vi "MattesImageRegistration.vi"(6 "Registration parameters":T1={"Sampling Percentage"=0.2, "maximum iteration"=200, "number of bins"=200}, 8 "error in (no error)":errorcluster, 9 "False color image in":T2, 10 "Moving image in":T2=refnum, 11 "Fixed image in":T2=refnum) -> (0 "error out":errorcluster, 1 "False color alignment image":T2, 2 "Moving image out (duplicate)":T2, 3 "Fixed image out (duplicate)":T2, 4 "alignment quality":dbl=-0.39635115330155946, 5 "y translation":dbl=4.5810062720041405, 7 "x translation":dbl=-23.66339978067731)   [LabVIEW 2012]
uses:
  <vilib>/vision/Image Controls.llb/IMAQ Image.ctl
  <vilib>/vision/NI_Vision_Development_Module.lvlib
  C++/bin/Release/ImageReg.dll
panel:
  out "elapsed time (ms)":u32=741
  out "# of iterations":dbl=100.0
  out "False color image":T2(plugin-control)
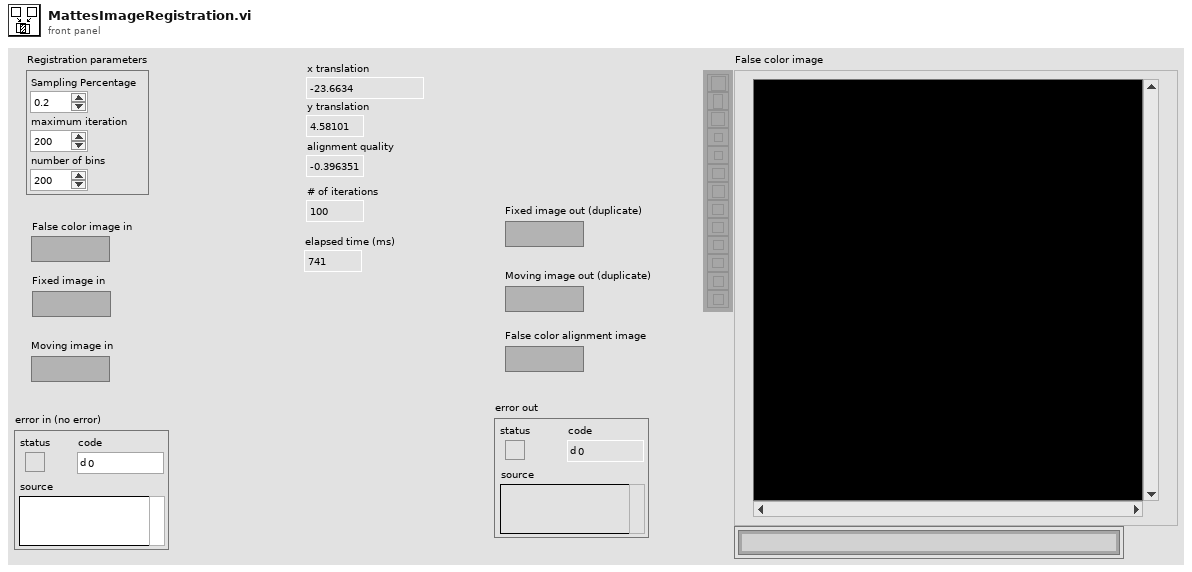
[diagram p1: front panel]
types:
  T1 = cluster{"Sampling Percentage":dbl, "maximum iteration":i32, "number of bins":u32}
  T2 = typedef "IMAQ Image.ctl" = refnum<image>
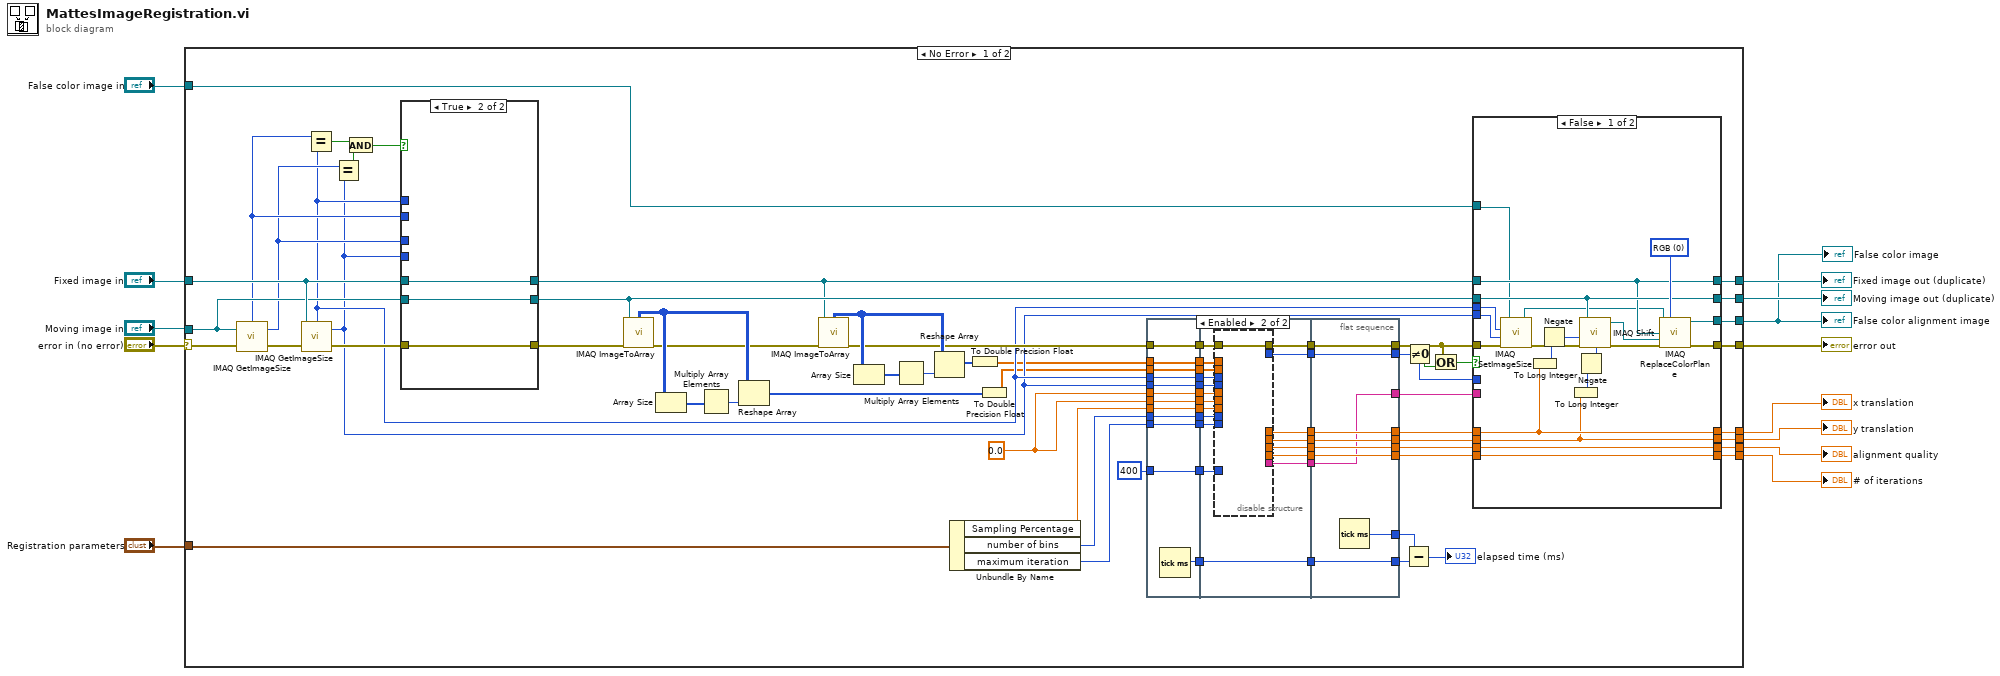
[diagram p0: block diagram]
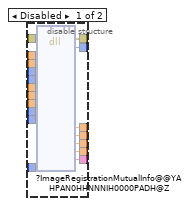
[diagram p2: hidden frame]
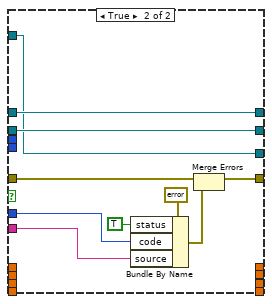
[diagram p3: hidden frame]
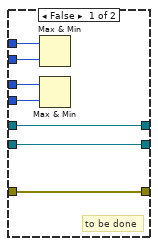
[diagram p4: hidden frame]
diagram:
  n1 = case shown="No Error" "error in (no error)" {
    selector: "error in (no error)" -> [w87 w191]
    tunnel: [w74 w191] -> w12
    tunnel: "Moving image in" -> [w81 w189]
    tunnel: "Fixed image in" -> [w82 w190]
    tunnel: [w67 _] -> w9
    tunnel: [w66 _] -> w8
    tunnel: [w65 _] -> w7
    tunnel: [w64 w188] -> w4
    tunnel: [w63 w189] -> w6
    tunnel: [w62 w190] -> w5
    tunnel: [w61 _] -> w3
    tunnel: "False color image in" -> [w30 w188]
    tunnel: "Registration parameters" -> [w27 _]
    frame No Error {
      w19 = 0.0 ("double precision float")
      n2 = call "IMAQ GetImageSize"("Image"=w81, "error in (no error)"=w87) -> ("Y Resolution"=w79:i32, "X Resolution"=w80:i32, "error out"=w86:errorcluster)  [unwired: 2 in]
      n3 = call "IMAQ GetImageSize"("Image"=w82, "error in (no error)"=w86) -> ("Y Resolution"=w57:i32, "X Resolution"=w58:i32, "error out"=w78:errorcluster)  [unwired: 2 in]
      n4 = Equal?(x=w80, y=w58) -> (x = y?=w84:bool)
      n5 = Equal?(x=w79, y=w57) -> (x = y?=w85:bool)
      n6 = And(x=w84, y=w85) -> (x .and. y?=w83:bool)
      n7 = case shown="True" w83 {
        tunnel: [w180 w187] -> w28
        tunnel: w82 -> [w180 w187]
        tunnel: [w179 w186] -> w29
        tunnel: w81 -> [w179 w186]
        tunnel: w58 -> [w184 _]
        tunnel: w80 -> [w183 _]
        tunnel: w79 -> [w182 _]
        tunnel: w57 -> [w181 _]
        tunnel: [w178 w185] -> w18
        tunnel: w78 -> [w178 w185]
        frame False {
          # "to be done"
          n8 = Max & Min(x=w184, y=w183) -> ()  [unwired: 2 out]
          n9 = Max & Min(x=w182, y=w181) -> ()  [unwired: 2 out]
        }
        frame True {
        }
      }
      n10 = call "IMAQ ImageToArray"("error in (no error)"=w18, "Image"=w29) -> ("error out"=w17:errorcluster, "Image Pixels (U8)"=w73:u8[][])  [unwired: 2 in, 3 out]
      n11 = Array Size(array=w73) -> (size(s)=w72:i32[])
      n12 = Multiply Array Elements(1:w72) -> (0:w71:i32)
      n13 = Reshape Array(w73, w71) -> (w77:u8[])
      n14 = call "IMAQ ImageToArray"("error in (no error)"=w17, "Image"=w28) -> ("error out"=w60:errorcluster, "Image Pixels (U8)"=w68:u8[][])  [unwired: 2 in, 3 out]
      n15 = Array Size(array=w68) -> (size(s)=w70:i32[])
      n16 = Multiply Array Elements(1:w70) -> (0:w69:i32)
      n17 = Reshape Array(w68, w69) -> (w21:u8[])
      n18 = Unbundle By Name(w27) -> ("Sampling Percentage"=w26:dbl, "number of bins"=w25:u32, "maximum iteration"=w16:i32)
      n19 = To Double Precision Float(number=w21) -> (double precision float=w20:dbl[])
      n20 = To Double Precision Float(number=w77) -> (double precision float=w22:dbl[])
      n21 = flat-sequence {
        tunnel: w26 -> [w92]
        tunnel: w19 -> [w93]
        tunnel: w19 -> [w94]
        tunnel: w57 -> [w95]
        tunnel: w58 -> [w96]
        tunnel: w22 -> [w97]
        tunnel: w20 -> [w98]
        tunnel: w60 -> [w99]
        tunnel: [w99] -> w51
        tunnel: [w98] -> w50
        tunnel: [w97] -> w49
        tunnel: [w96] -> w48
        tunnel: [w95] -> w47
        tunnel: [w94] -> w46
        tunnel: [w93] -> w45
        tunnel: [w92] -> w44
        tunnel: [w91] -> w36
        tunnel: [w90] -> w32
        tunnel: w16 -> [w90]
        tunnel: [w89] -> w31
        tunnel: w25 -> [w89]
        tunnel: 400 ("dimension size") -> [w88]
        tunnel: [w88] -> w14
        tunnel: w51 -> [w118]
        tunnel: w50 -> [w116]
        tunnel: w49 -> [w115]
        tunnel: w48 -> [w114]
        tunnel: w47 -> [w113]
        tunnel: w46 -> [w112]
        tunnel: w45 -> [w111]
        tunnel: w44 -> [w110]
        tunnel: [w117] -> w43
        tunnel: [w109] -> w42
        tunnel: [w108] -> w41
        tunnel: [w107] -> w40
        tunnel: [w106] -> w39
        tunnel: [w105] -> w38
        tunnel: w36 -> [w104]
        tunnel: [w104] -> w35
        tunnel: w32 -> [w103]
        tunnel: w31 -> [w102]
        tunnel: [w101] -> w23
        tunnel: w14 -> [w100]
        tunnel: [w141] -> w52
        tunnel: [w142] -> w53
        tunnel: [w143] -> w54
        tunnel: [w144] -> w55
        tunnel: [w145] -> w56
        tunnel: [w146] -> w59
        tunnel: w43 -> [w146]
        tunnel: w42 -> [w145]
        tunnel: w41 -> [w144]
        tunnel: w40 -> [w143]
        tunnel: w39 -> [w142]
        tunnel: w38 -> [w141]
        tunnel: [w140] -> w37
        tunnel: w35 -> [w139]
        tunnel: [w139] -> w34
        tunnel: [w138] -> w24
        tunnel: w23 -> [w138]
        frame #0 {
          n22 = Tick Count (ms)() -> (millisecond timer value=w91:u32)
        }
        frame #1 {
          n23 = disable-structure shown="Enabled" {
            disable-tunnel: w118 -> [w136 w137]
            disable-tunnel: [w135 w137] -> w117
            disable-tunnel: w116 -> [w134 _]
            disable-tunnel: w115 -> [w133 _]
            disable-tunnel: w114 -> [w132 _]
            disable-tunnel: w113 -> [w131 _]
            disable-tunnel: w112 -> [w130 _]
            disable-tunnel: w111 -> [w129 _]
            disable-tunnel: w110 -> [w128 _]
            disable-tunnel: [w127 _] -> w109
            disable-tunnel: [w126 _] -> w108
            disable-tunnel: [w125 _] -> w107
            disable-tunnel: [w124 _] -> w106
            disable-tunnel: [w123 _] -> w105
            disable-tunnel: w103 -> [w122 _]
            disable-tunnel: w102 -> [w121 _]
            disable-tunnel: [w120 _] -> w101
            disable-tunnel: w100 -> [w119 _]
            frame Disabled {
              n24 = dll-call lib="D:/Moroder/dependencies/ImageReg/C++/bin/Release/ImageReg.dll" fn="?ImageRegistrationMutualInfo@@YAHPAN0HHNNNIH0000PADH@Z"(error in=w136, "fixed image"=w134, "moving image"=w133, "image width"=w132, "image height"=w131, "initial x translation"=w130, "initial y translation"=w129, "sampling percentage"=w128, "number of bins"=w121, "maximum iteration"=w122, "errlength"=w119) -> (error out=w135:errorcluster, "error flag"=w123:i32, "x translation"=w127:dbl, "y translation"=w126:dbl, "quality"=w125:dbl, "number of iterations"=w124:dbl, "error"=w120:string)  [unwired: 17 in, 1 out]
            }
            frame Enabled {
            }
          }
        }
        frame #2 {
          n25 = Tick Count (ms)() -> (millisecond timer value=w140:u32)
        }
      }
      n26 = Subtract(x=w37, y=w34) -> (x-y=→"elapsed time (ms)":u32)
      n27 = Not Equal To 0?(x=w52) -> (x != 0?=w76:bool)
      n28 = Or(x=w59, y=w76) -> (x .or. y?=w75:bool)
      n29 = case shown="False" w75 {
        tunnel: w59 -> [w148 w173]
        tunnel: w52 -> [_ w176]
        tunnel: [w164 w172] -> w74
        tunnel: w29 -> [w158 w169]
        tunnel: w56 -> [w162 _]
        tunnel: w55 -> [w161 _]
        tunnel: w28 -> [w157 w170]
        tunnel: [w162 _] -> w67
        tunnel: [w161 _] -> w66
        tunnel: [w160 _] -> w65
        tunnel: w54 -> [w160 _]
        tunnel: [w159 w168] -> w64
        tunnel: [w158 w169] -> w63
        tunnel: [w157 w170] -> w62
        tunnel: [w152 _] -> w61
        tunnel: w53 -> [w152 _]
        tunnel: w58 -> [w150 _]
        tunnel: w57 -> [w149 _]
        tunnel: w30 -> [w147 w168]
        tunnel: w24 -> [_ w171]
        frame False {
          w163 = u16 0 items=["RGB", "HSL", "HSV", "HSI"] ("Color Mode")
          n30 = call "IMAQ SetImageSize"("error in (no error)"=w148, "Y Resolution"=w149, "X Resolution"=w150, "Image"=w147) -> ("error out"=w151:errorcluster, "Image Out"=w155:T2)  [unwired: 1 in]
          n31 = To Long Integer(number=w162) -> (32bit integer=w167:i32)
          n32 = Negate(x=w167) -> (-x=w154:i32)
          n33 = To Long Integer(number=w161) -> (32bit integer=w166:i32)
          n34 = Negate(x=w166) -> (-x=w153:i32)
          n35 = call "IMAQ Shift"("YOffset"=w153, "error in (no error)"=w151, "XOffset"=w154, "Image Src"=w158) -> ("error out"=w165:errorcluster, "Image Dst Out"=w156:T2)  [unwired: 6 in]
          n36 = call "IMAQ ReplaceColorPlane"("Image Src"=w155, "Color Mode"=w163, "Red or Hue Plane"=w157, "Green or Sat Plane"=w156, "error in (no error)"=w165) -> ("Image Dst Out"=w159:T2, "error out"=w164:errorcluster)  [unwired: 9 in]
        }
        frame True {
          n37 = Bundle By Name(cluster=errorcluster {"status"=FALSE, "code"=0, "source"=""} ("error in"), "status"=TRUE, "code"=w176, "source"=w171) -> (w174:errorcluster)
          n38 = Merge Errors(w173, w174) -> (w172:errorcluster)
        }
      }
    }
    frame Error {
    }
  }
  "error out" <- w12
  "x translation" <- w9
  "y translation" <- w8
  "alignment quality" <- w7
  "Fixed image out (duplicate)" <- w5
  "Moving image out (duplicate)" <- w6
  "False color alignment image" <- w4
  "False color image" <- w4
  "# of iterations" <- w3
